vi "R1DataCollection.vi"(8 "error constant":errorcluster, 10 "Write Once":bool, 11 "LabVIEW Web Service":refnum<class "Web Service.lvclass">) -> (0 "error out":errorcluster={"status"=FALSE, "code"=0, "source"="0"})   [LabVIEW 2016]
uses:
  <vilib>/wsapi/Web Service.lvclass
  <vilib>/Platform/TimedLoop/XDataNode/timing_clust.ctl
  <vilib>/Platform/TimedLoop/XDataNode/nitl_modes.ctl
  <vilib>/Platform/TimedLoop/XDataNode/wakeup.ctl
  <vilib>/Platform/TimedLoop/XDataNode/XDataNode.xnode
  <vilib>/Platform/TimedLoop/XDataNode/XDNodeRunTimeDep.lvlib
  <vilib>/ptbypt/NI_PtbyPt.lvlib
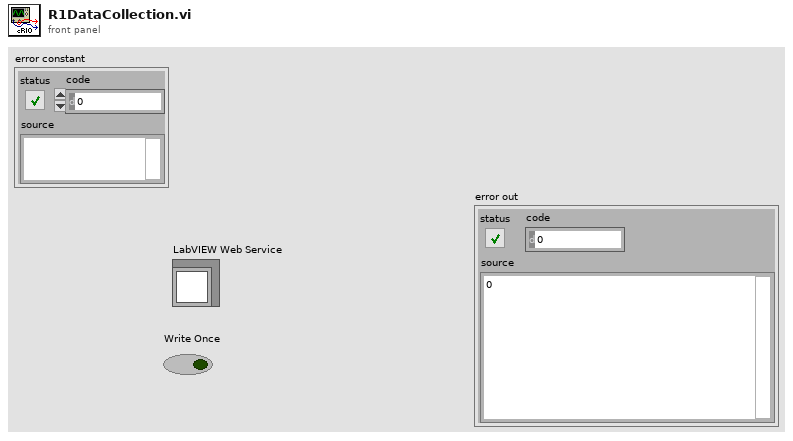
[diagram p1: front panel]
types:
  T1 = typedef "XDNodeRunTimeDep.lvlib/timing_clust.ctl" = cluster{"Expected End [f-1]":u64, "Actual End [f-1]":u64, "Finished Late? [f-1]":bool, "Expected End [i-1]":u64, "Actual End [i-1]":u64, "Finished Late? [i-1]":bool, "Expected Start [i]":u64, "Actual Start [i]":u64, "Expected Start [f]":u64, "Actual Start [f]":u64, "Source Name":string, "Structure Name":string, "Period":i64, "Deadline":i64, "Offset":i64, "Start":i64, "Priority":i32, "Timeout":i32, "Mode":T2, "Wakeup Reason":T3, "Error":errorcluster, "Source Type":string, "Secondary Source Type":string, "Global End Time":u64, "Global Start Time":u64, "Frame Duration":u64, "Iteration Duration":u64, "Assigned CPU":i32, "I/O Scan Engine Mode":u32}
  T2 = typedef "XDNodeRunTimeDep.lvlib/nitl_modes.ctl" = enum32{"No Change", "Process missed periods, maintain original phase", "Discard missed periods, maintain original phase", "Process missed periods, ignore original phase", "Discard missed periods, ignore original phase"}
  T3 = typedef "XDNodeRunTimeDep.lvlib/wakeup.ctl" = enum32{"Normal", "Aborted", "Asynchronous wakeup", "Timing source error", "Timed loop error", "Timeout"}
  T4 = cluster{"Media Pump":bool, "Water Pump":bool, "Gas Pump":bool, "Effluent Pump":bool}
  T5 = cluster{"Array of Double[0]":dbl, "Array of Double[1]":dbl, "Array of Double[2]":dbl, "Array of Double[3]":dbl, "Array of Double[4]":dbl, "Array of Double[5]":dbl, "Array of Double[6]":dbl, "Array of Double[7]":dbl, "Array of Double[8]":dbl}
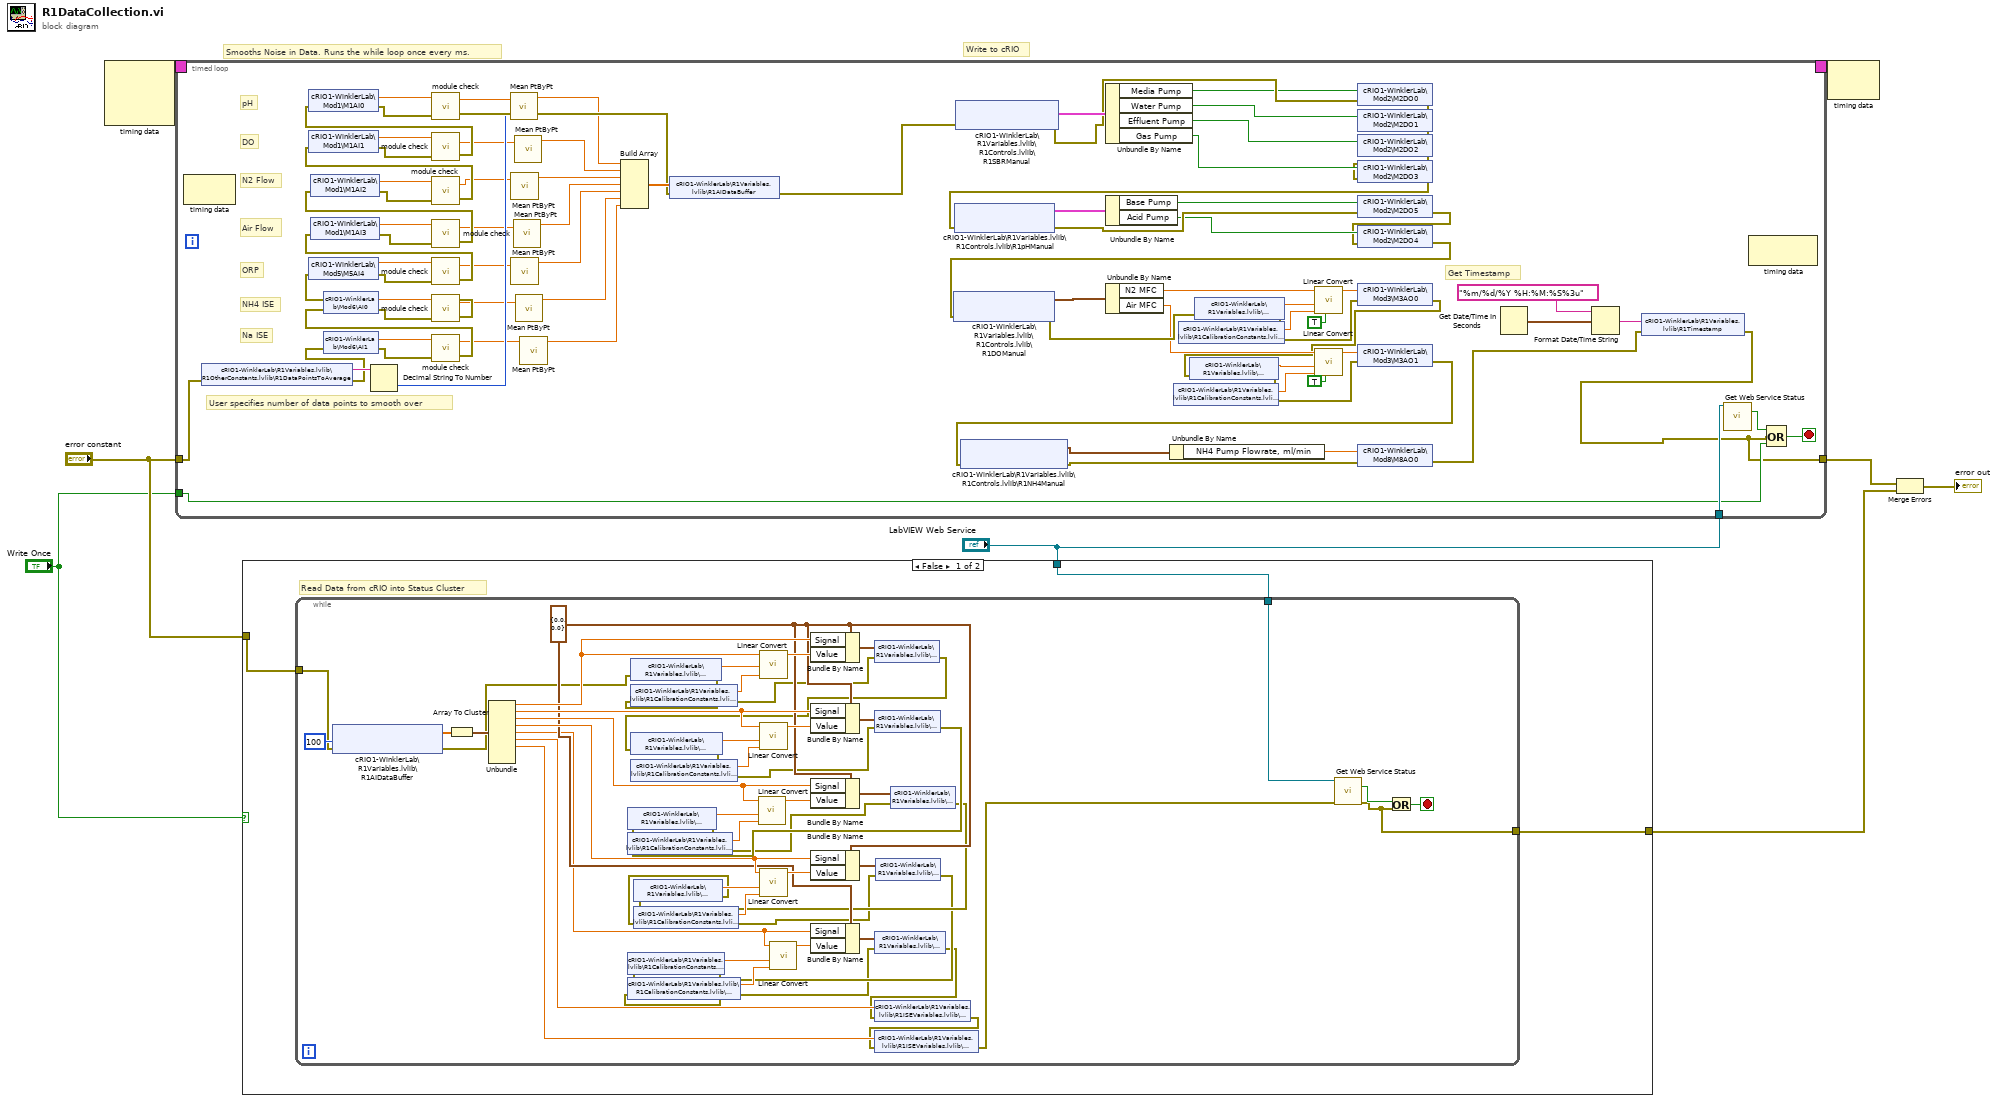
[diagram p0: block diagram]
diagram:
  # "Write to cRIO"
  # "Smooths Noise in Data. Runs the while loop once every ms."
  n1 = node-c288() -> (w8:T1)  [unwired: 3 in]
  n2 = timed-loop {
    timing: w8 -> [_]
    timing-out: [_] -> w7
    tunnel: "error constant" -> [w83]
    tunnel: "LabVIEW Web Service" -> [w76]
    tunnel: "Write Once" -> [w74]
    tunnel: [w73] -> w3
    stop <- w72 stop-if-true
    # "NH4 ISE"
    # "Na ISE"
    # "ORP"
    # "Get Timestamp"
    # "User specifies number of data points to smooth over"
    # "Air Flow"
    # "N2 Flow"
    # "DO"
    # "pH"
    n3 = node-c288() -> ()  [unwired: 1 in, 1 out]
    n4 = shared-variable "cRIO1-WinklerLab\\R1Variables.lvlib\\R1OtherConstants.lvlib\\R1DataPointsToAverage"(error in=w83) -> (w91:string, error out=w67:errorcluster)
    n5 = shared-variable "cRIO1-WinklerLab\\Mod6\\AI1"(error in=w67) -> (w71:dbl, error out=w70:errorcluster)
    n6 = Decimal String To Number(string=w91) -> (number=w49:i32)  [unwired: 2 in, 1 out]
    n7 = call "module check.vi"("error in"=w70, "Value"=w71) -> ("error constant"=w68:errorcluster, "Value out"=w46:dbl)  [unwired: 1 in]
    n8 = shared-variable "cRIO1-WinklerLab\\Mod6\\AI0"(error in=w68) -> (w69:dbl, error out=w66:errorcluster)
    n9 = call "module check.vi"("error in"=w66, "Value"=w69) -> ("error constant"=w65:errorcluster, "Value out"=w44:dbl)  [unwired: 1 in]
    n10 = shared-variable "cRIO1-WinklerLab\\Mod5\\M5AI4"(error in=w65) -> (w64:dbl, error out=w63:errorcluster)
    n11 = call "module check.vi"("error in"=w63, "Value"=w64) -> ("error constant"=w62:errorcluster, "Value out"=w42:dbl)  [unwired: 1 in]
    n12 = shared-variable "cRIO1-WinklerLab\\Mod1\\M1AI3"(error in=w62) -> (w61:dbl, error out=w60:errorcluster)
    n13 = call "module check.vi"("error in"=w60, "Value"=w61) -> ("error constant"=w59:errorcluster, "Value out"=w39:dbl)  [unwired: 1 in]
    n14 = shared-variable "cRIO1-WinklerLab\\Mod1\\M1AI2"(error in=w59) -> (w58:dbl, error out=w57:errorcluster)
    n15 = call "module check.vi"("error in"=w57, "Value"=w58) -> ("error constant"=w56:errorcluster, "Value out"=w38:dbl)  [unwired: 1 in]
    n16 = shared-variable "cRIO1-WinklerLab\\Mod1\\M1AI1"(error in=w56) -> (w54:dbl, error out=w55:errorcluster)
    n17 = call "module check.vi"("error in"=w55, "Value"=w54) -> ("error constant"=w52:errorcluster, "Value out"=w35:dbl)  [unwired: 1 in]
    n18 = shared-variable "cRIO1-WinklerLab\\Mod1\\M1AI0"(error in=w52) -> (w53:dbl, error out=w51:errorcluster)
    n19 = call "module check.vi"("error in"=w51, "Value"=w53) -> ("error constant"=w50:errorcluster, "Value out"=w48:dbl)  [unwired: 1 in]
    n20 = call <vilib>:"Mean PtByPt.vi"("x"=w48, "sample length"=w49) -> ("mean"=w47:dbl)  [unwired: 2 in, 1 out]
    n21 = call <vilib>:"Mean PtByPt.vi"("x"=w38) -> ("mean"=w37:dbl)  [unwired: 3 in, 1 out]
    n22 = call <vilib>:"Mean PtByPt.vi"("x"=w42) -> ("mean"=w41:dbl)  [unwired: 3 in, 1 out]
    n23 = call <vilib>:"Mean PtByPt.vi"("x"=w39) -> ("mean"=w40:dbl)  [unwired: 3 in, 1 out]
    n24 = call <vilib>:"Mean PtByPt.vi"("x"=w35) -> ("mean"=w36:dbl)  [unwired: 3 in, 1 out]
    n25 = call <vilib>:"Mean PtByPt.vi"("x"=w44) -> ("mean"=w43:dbl)  [unwired: 3 in, 1 out]
    n26 = call <vilib>:"Mean PtByPt.vi"("x"=w46) -> ("mean"=w45:dbl)  [unwired: 3 in, 1 out]
    n27 = Build Array(w47, w36, w37, w40, w41, w43, w45) -> (w95:dbl[])
    n28 = shared-variable "cRIO1-WinklerLab\\R1Variables.lvlib\\R1AIDataBuffer"(w95, error in=w50) -> (error out=w82:errorcluster)
    n29 = shared-variable "cRIO1-WinklerLab\\R1Variables.lvlib\\R1Controls.lvlib\\R1SBRManual"(error in=w82) -> (w90:T4, error out=w81:errorcluster)  [unwired: 1 in, 1 out]
    n30 = Unbundle By Name(w90) -> ("Media Pump"=w34:bool, "Water Pump"=w32:bool, "Effluent Pump"=w33:bool, "Gas Pump"=w31:bool)
    n31 = shared-variable "cRIO1-WinklerLab\\Mod2\\M2DO0"(w34, error in=w81) -> (error out=w28:errorcluster)
    n32 = shared-variable "cRIO1-WinklerLab\\Mod2\\M2DO1"(w32, error in=w28) -> (error out=w29:errorcluster)
    n33 = shared-variable "cRIO1-WinklerLab\\Mod2\\M2DO2"(w33, error in=w29) -> (error out=w30:errorcluster)
    n34 = shared-variable "cRIO1-WinklerLab\\Mod2\\M2DO3"(w31, error in=w30) -> (error out=w87:errorcluster)
    n35 = shared-variable "cRIO1-WinklerLab\\R1Variables.lvlib\\R1Controls.lvlib\\R1pHManual"(error in=w87) -> (w89:cluster{"Acid Pump":bool, "Base Pump":bool}, error out=w86:errorcluster)  [unwired: 1 in, 1 out]
    n36 = Unbundle By Name(w89) -> ("Base Pump"=w26:bool, "Acid Pump"=w27:bool)
    n37 = shared-variable "cRIO1-WinklerLab\\Mod2\\M2DO5"(w26, error in=w86) -> (error out=w25:errorcluster)
    n38 = shared-variable "cRIO1-WinklerLab\\Mod2\\M2DO4"(w27, error in=w25) -> (error out=w77:errorcluster)
    n39 = shared-variable "cRIO1-WinklerLab\\R1Variables.lvlib\\R1Controls.lvlib\\R1DOManual"(error in=w77) -> (w79:cluster{"Air MFC":dbl, "N2 MFC":dbl}, error out=w78:errorcluster)  [unwired: 1 in, 1 out]
    n40 = Unbundle By Name(w79) -> ("N2 MFC"=w23:dbl, "Air MFC"=w22:dbl)
    n41 = shared-variable "cRIO1-WinklerLab\\R1Variables.lvlib\\R1CalibrationConstants.lvlib\\R1N2Slope"(error in=w78) -> (w17:dbl, error out=w14:errorcluster)
    n42 = shared-variable "cRIO1-WinklerLab\\R1Variables.lvlib\\R1CalibrationConstants.lvlib\\R1N2Intercept"(error in=w14) -> (w16:dbl, error out=w13:errorcluster)
    n43 = call "Linear Convert.vi"("Inverse?"=TRUE, "Intercept"=w16, "Slope"=w17, "Signal"=w23) -> ("Result"=w15:dbl)  [unwired: 7 in]
    n44 = shared-variable "cRIO1-WinklerLab\\Mod3\\M3AO0"(w15, error in=w13) -> (error out=w12:errorcluster)
    n45 = shared-variable "cRIO1-WinklerLab\\R1Variables.lvlib\\R1CalibrationConstants.lvlib\\R1AirSlope"(error in=w12) -> (w19:dbl, error out=w11:errorcluster)
    n46 = shared-variable "cRIO1-WinklerLab\\R1Variables.lvlib\\R1CalibrationConstants.lvlib\\R1AirIntercept"(error in=w11) -> (w18:dbl, error out=w10:errorcluster)
    n47 = call "Linear Convert.vi"("Inverse?"=TRUE, "Intercept"=w18, "Slope"=w19, "Signal"=w22) -> ("Result"=w24:dbl)  [unwired: 7 in]
    n48 = shared-variable "cRIO1-WinklerLab\\Mod3\\M3AO1"(w24, error in=w10) -> (error out=w85:errorcluster)
    n49 = shared-variable "cRIO1-WinklerLab\\R1Variables.lvlib\\R1Controls.lvlib\\R1NH4Manual"(error in=w85) -> (w88:cluster{"NH4 Pump Flowrate, ml/min":dbl}, error out=w84:errorcluster)  [unwired: 1 in, 1 out]
    n50 = Unbundle By Name(w88) -> ("NH4 Pump Flowrate, ml/min"=w9:dbl)
    n51 = shared-variable "cRIO1-WinklerLab\\Mod8\\M8AO0"(w9, error in=w84) -> (error out=w80:errorcluster)
    n52 = Get Date/Time In Seconds() -> (seconds since 1Jan1904=w93:timestamp)
    n53 = Format Date/Time String(time format string (%c)="%m/%d/%Y %H:%M:%S%3u", seconds (now)=w93) -> (date/time string=w92:string)  [unwired: 1 in]
    n54 = shared-variable "cRIO1-WinklerLab\\R1Variables.lvlib\\R1Timestamp"(w92, error in=w80) -> (error out=w73:errorcluster)
    n55 = call <vilib>:"Get Web Service Status.vi"("LabVIEW Web Service"=w76) -> ("service stopping?"=w75:bool)  [unwired: 12 in, 2 out]
    n56 = node-c288() -> ()  [unwired: 1 in, 1 out]
    n57 = Compound Arithmetic op=OR(w75, w73, w74) -> (w72:bool)
  }
  n58 = case shown="False" "Write Once" {
    tunnel: "error constant" -> [w100 w155]
    tunnel: "LabVIEW Web Service" -> [w99 _]
    tunnel: [w98 w155] -> w2
    frame False {
      # "Read Data from cRIO into Status Cluster"
      n59 = while {
        tunnel: w100 -> [w104]
        tunnel: [w102] -> w98
        tunnel: w99 -> [w101]
        stop <- w144 stop-if-true
        w131 = cluster{"Signal":dbl, "Value":dbl} {"Signal"=0.0, "Value"=0.0} ("Analog Input")
        n60 = shared-variable "cRIO1-WinklerLab\\R1Variables.lvlib\\R1AIDataBuffer"(error in=w104, u32 100 ("milliseconds to wait")) -> (w152:dbl[], error out=w121:errorcluster)  [unwired: 1 out]
        n61 = Array To Cluster(array=w152) -> (cluster=w154:T5)
        n62 = Unbundle(w154) -> ("Array of Double[0]"=w150:dbl, "Array of Double[1]"=w148:dbl, "Array of Double[2]"=w137:dbl, "Array of Double[3]"=w136:dbl, "Array of Double[4]"=w128:dbl, "Array of Double[5]"=w135:dbl, "Array of Double[6]"=w134:dbl)  [unwired: 2 out]
        n63 = shared-variable "cRIO1-WinklerLab\\R1Variables.lvlib\\R1CalibrationConstants.lvlib\\R1pHSlope"(error in=w121) -> (w142:dbl, error out=w120:errorcluster)
        n64 = shared-variable "cRIO1-WinklerLab\\R1Variables.lvlib\\R1CalibrationConstants.lvlib\\R1pHIntercept"(error in=w120) -> (w143:dbl, error out=w119:errorcluster)
        n65 = call "Linear Convert.vi"("Intercept"=w143, "Slope"=w142, "Signal"=w150) -> ("Result"=w151:dbl)  [unwired: 8 in]
        n66 = Bundle By Name(cluster=w131, "Signal"=w150, "Value"=w151) -> (w149:cluster{"Signal":dbl, "Value":dbl})
        n67 = shared-variable "cRIO1-WinklerLab\\R1Variables.lvlib\\R1Signals.lvlib\\R1pH"(w149, error in=w119) -> (error out=w118:errorcluster)
        n68 = shared-variable "cRIO1-WinklerLab\\R1Variables.lvlib\\R1CalibrationConstants.lvlib\\R1DOSlope"(error in=w118) -> (w141:dbl, error out=w117:errorcluster)
        n69 = shared-variable "cRIO1-WinklerLab\\R1Variables.lvlib\\R1CalibrationConstants.lvlib\\R1DOIntercept"(error in=w117) -> (w140:dbl, error out=w116:errorcluster)
        n70 = call "Linear Convert.vi"("Intercept"=w140, "Slope"=w141, "Signal"=w148) -> ("Result"=w146:dbl)  [unwired: 8 in]
        n71 = Bundle By Name(cluster=w131, "Signal"=w148, "Value"=w146) -> (w147:cluster{"Signal":dbl, "Value":dbl})
        n72 = shared-variable "cRIO1-WinklerLab\\R1Variables.lvlib\\R1Signals.lvlib\\R1DO"(w147, error in=w116) -> (error out=w115:errorcluster)
        n73 = shared-variable "cRIO1-WinklerLab\\R1Variables.lvlib\\R1CalibrationConstants.lvlib\\R1N2Slope"(error in=w115) -> (w125:dbl, error out=w114:errorcluster)
        n74 = shared-variable "cRIO1-WinklerLab\\R1Variables.lvlib\\R1CalibrationConstants.lvlib\\R1N2Intercept"(error in=w114) -> (w124:dbl, error out=w113:errorcluster)
        n75 = call "Linear Convert.vi"("Intercept"=w124, "Slope"=w125, "Signal"=w137) -> ("Result"=w138:dbl)  [unwired: 8 in]
        n76 = Bundle By Name(cluster=w131, "Signal"=w137, "Value"=w138) -> (w122:cluster{"Signal":dbl, "Value":dbl})
        n77 = shared-variable "cRIO1-WinklerLab\\R1Variables.lvlib\\R1Signals.lvlib\\R1N2"(w122, error in=w113) -> (error out=w112:errorcluster)
        n78 = shared-variable "cRIO1-WinklerLab\\R1Variables.lvlib\\R1CalibrationConstants.lvlib\\R1AirSlope"(error in=w112) -> (w127:dbl, error out=w111:errorcluster)
        n79 = shared-variable "cRIO1-WinklerLab\\R1Variables.lvlib\\R1CalibrationConstants.lvlib\\R1AirIntercept"(error in=w111) -> (w126:dbl, error out=w110:errorcluster)
        n80 = call "Linear Convert.vi"("Intercept"=w126, "Slope"=w127, "Signal"=w136) -> ("Result"=w139:dbl)  [unwired: 8 in]
        n81 = Bundle By Name(cluster=w131, "Signal"=w136, "Value"=w139) -> (w123:cluster{"Signal":dbl, "Value":dbl})
        n82 = shared-variable "cRIO1-WinklerLab\\R1Variables.lvlib\\R1Signals.lvlib\\R1Air"(w123, error in=w110) -> (error out=w109:errorcluster)
        n83 = shared-variable "cRIO1-WinklerLab\\R1Variables.lvlib\\R1CalibrationConstants.lvlib\\R1ORPSlope"(error in=w109) -> (w130:dbl, error out=w108:errorcluster)
        n84 = shared-variable "cRIO1-WinklerLab\\R1Variables.lvlib\\R1CalibrationConstants.lvlib\\R1ORPIntercept"(error in=w108) -> (w129:dbl, error out=w107:errorcluster)
        n85 = call "Linear Convert.vi"("Intercept"=w129, "Slope"=w130, "Signal"=w128) -> ("Result"=w133:dbl)  [unwired: 8 in]
        n86 = Bundle By Name(cluster=w131, "Signal"=w128, "Value"=w133) -> (w132:cluster{"Signal":dbl, "Value":dbl})
        n87 = shared-variable "cRIO1-WinklerLab\\R1Variables.lvlib\\R1Signals.lvlib\\R1ORP"(w132, error in=w107) -> (error out=w106:errorcluster)
        n88 = shared-variable "cRIO1-WinklerLab\\R1Variables.lvlib\\R1ISEVariables.lvlib\\R1NaISERaw"(w135, error in=w106) -> (error out=w105:errorcluster)
        n89 = shared-variable "cRIO1-WinklerLab\\R1Variables.lvlib\\R1ISEVariables.lvlib\\R1NH4ISERaw"(w134, error in=w105) -> (error out=w103:errorcluster)
        n90 = call <vilib>:"Get Web Service Status.vi"("LabVIEW Web Service"=w101, "error in (no error)"=w103) -> ("service stopping?"=w145:bool, "error out"=w102:errorcluster)  [unwired: 11 in, 1 out]
        n91 = Or(x=w145, y=w102) -> (x .or. y?=w144:bool)
      }
    }
    frame True {
    }
  }
  n92 = node-c288(w7) -> ()  [unwired: 1 out]
  n93 = Merge Errors(w3, w2) -> (→"error out":errorcluster)
